vi "_RT_CtrlLoop_Reboot_Monitor.vi"(8 "error in (no error)":errorcluster) -> ()   [LabVIEW 2018]
uses:
  PublicSubVI/Ctl/_ctl_RT_Working_State.ctl
  PublicSubVI/Ctl/_ctl_RT_SysLog.ctl
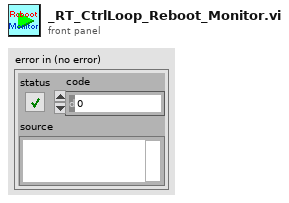
[diagram p1: front panel]
types:
  T1 = typedef "_ctl_RT_SysLog.ctl" = enum16{"None", "Initialize", "StartupRT", "StartupFPGA", "StartupAllocator", "GetMass", "SetWfmCode", "SetLaserCtrl", "SetTurboCtrl", "SetD999Ctrl", "Reconnecting...", "Interrupt", "StopRT"}
  T2 = typedef "_ctl_RT_Working_State.ctl" = enum16{"Initialize", "Running", "Reboot_Work", "Reboot_Safe"}
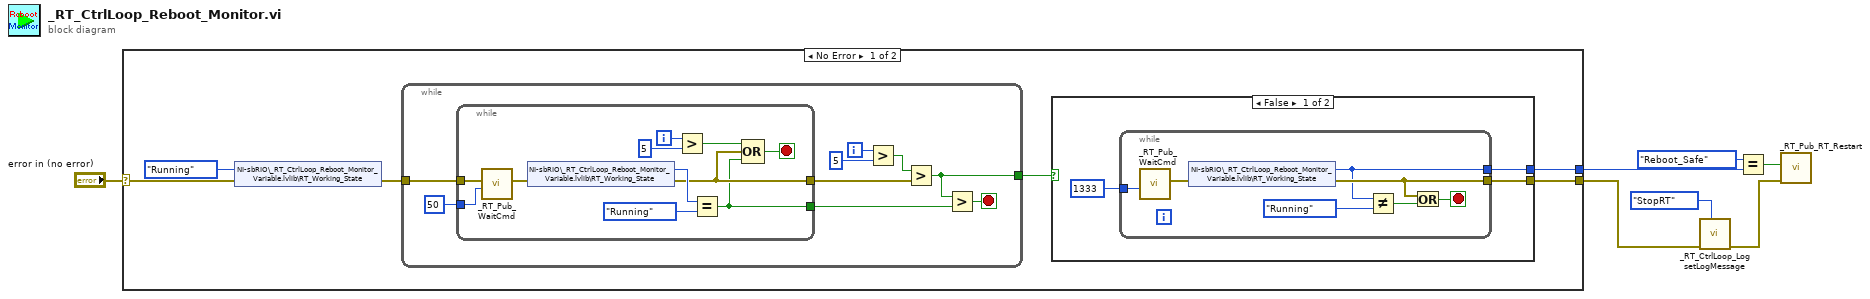
[diagram p0: block diagram]
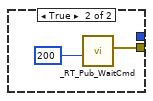
[diagram p2: hidden frame]
diagram:
  n1 = case shown="No Error" "error in (no error)" {
    selector: "error in (no error)" -> [w9 w46]
    tunnel: [w13 w46] -> w3
    tunnel: [w12 _] -> w7
    frame No Error {
      n2 = shared-variable "NI-sbRIO\\_RT_CtrlLoop_Reboot_Monitor_Variable.lvlib\\RT_Working_State"(_ctl_RT_Working_State."Running" ("RT_Working_State"), error in=w9) -> (error out=w8:errorcluster)
      n3 = while {
        tunnel: w8 -> [w14]
        tunnel: [w17] -> w11
        i -> [w21]
        stop <- w15 stop-if-true
        n4 = while {
          tunnel: w14 -> [w29]
          tunnel: [w25] -> w18
          tunnel: u32 50 ("milliseconds to wait") -> [w27]
          tunnel: [w24] -> w16
          i -> [w31]
          stop <- w23 stop-if-true
          n5 = call "_RT_Pub_WaitCmd.vi"("milliseconds to wait"=w27, "error in (no error)"=w29) -> ("error out"=w28:errorcluster)  [unwired: 9 in]
          n6 = shared-variable "NI-sbRIO\\_RT_CtrlLoop_Reboot_Monitor_Variable.lvlib\\RT_Working_State"(error in=w28) -> (w33:T2, error out=w25:errorcluster)
          n7 = Greater?(x=w31, y=5) -> (0:w26:bool)
          n8 = Equal?(x=w33, y=_ctl_RT_Working_State."Running") -> (x = y?=w24:bool)
          n9 = Compound Arithmetic op=OR(w26, w25, w24) -> (w23:bool)
        }
        n10 = Greater?(x=w21, y=5) -> (0:w19:bool)
        n11 = Greater?(x=w19, y=w18) -> (0:w17:bool)
        n12 = Greater?(x=w17, y=w16) -> (0:w15:bool)
      }
      n13 = case shown="False" w11 {
        tunnel: [w36 w45] -> w13
        tunnel: [w34 _] -> w12
        frame False {
          n14 = while {
            tunnel: [w41] -> w36
            tunnel: u32 1333 ("milliseconds to wait") -> [w38]
            tunnel: [w37] -> w34
            stop <- w39 stop-if-true
            n15 = call "_RT_Pub_WaitCmd.vi"("milliseconds to wait"=w38) -> ("error out"=w43:errorcluster)  [unwired: 10 in]
            n16 = shared-variable "NI-sbRIO\\_RT_CtrlLoop_Reboot_Monitor_Variable.lvlib\\RT_Working_State"(error in=w43) -> (w37:T2, error out=w41:errorcluster)
            n17 = Not Equal?(x=w37, y=_ctl_RT_Working_State."Running") -> (x != y?=w40:bool)
            n18 = Or(x=w41, y=w40) -> (x .or. y?=w39:bool)
          }
        }
        frame True {
          n19 = call "_RT_Pub_WaitCmd.vi"("milliseconds to wait"=u32 200) -> ("error out"=w45:errorcluster)  [unwired: 10 in]
        }
      }
    }
    frame Error {
    }
  }
  n20 = call "_RT_CtrlLoop_Log setLogMessage.vi"("system type"=_ctl_RT_SysLog."StopRT", "error in"=w3) -> ("error out"=w2:errorcluster)  [unwired: 8 in, 1 out]
  n21 = Equal?(x=_ctl_RT_Working_State."Reboot_Safe", y=w7) -> (x = y?=w5:bool)
  n22 = call "_RT_Pub_RT_Restart.vi"("error in (no error)"=w2, "Safe Mode?"=w5) -> ()  [unwired: 9 in, 1 out]
